vi "HighFrameRateRecording - DX cameras 2.vi"() -> ()   [LabVIEW 2010]
doc: "The LL Ring VI acquires images continuously and displays them in an image control using the low-level acquisition VIs. A ring initiates a continuous high-speed acquisition to multiple buffers and is appropriate for high-speed applications that perform processing on every image. Multiple buffers are useful when processing times vary depending on other applications and processing results .\n\nIMAQ Init initializes the device. IMAQ Configure List configures the buffer list with multiple buffers. IMAQ Create creates the image buffers. Call IMAQ Configure Buffer once for each buffer in the buffer list. IMAQ Start starts the acquisition, and IMAQ Extract Buffer ensures that the current image is not overwritten. An image control displays the image on the front panel. After exiting the loop, IMAQ Extract Buffer releases the last extracted buffer. IMAQ Close releases resources associated with the acquisition, and IMAQ Dispose frees the image buffer."
uses:
  <vilib>/vision/Avi.llb/IMAQ AVI2 Codec Path.ctl
  <vilib>/vision/driver/NI_Vision_Acquisition_Software.lvlib
  <vilib>/vision/driver/IMAQdx.llb/IMAQdx Acquisition Mode.ctl
  <vilib>/vision/driver/IMAQdx.llb/IMAQdx Buffer Number Mode.ctl
  <vilib>/vision/Avi.llb/IMAQ AVI2 Refnum.ctl
  <vilib>/userdefined/High Color/IMAQdx.ctl
panel:
  out "Frame Rate Graph":dbl(graph)=23.976023976023978
  out "FPS":dbl=24.7320692497939 format="%#.1f"
  in  "Camera Selection DX":T1="cam2"
  out "AVI Refnum":T2
  out "Video recording":bool
  in  "Record?":bool
  in  "codec index":i32=4
  out "codec":string="Motion JPEG (NI Vision)"
  in  "AVI File Path":path=path "E:/Video/24fps.avi"
  out "Processed Frames/s":dbl=23.976023976023978 format="%#.1g"
  in  "Stop":bool
  out "Saved Frames":i32
  out "Image":T3(plugin-control)
  # "ToDo:\n - add JSON output\n - andd indicator of _s# number"
  # "1.  Initialisation"
  # "Codec should be:\n\"Y800 Uncompressed Grey Scale\""
  # "Naming convention:\n - use the name above and add _s#.avi for videos\n - specs for saved videos is specified in name.json"
  # "2.  Recording"
  # "y"
  # "Record"
  # "x"
  # "Just Observe"
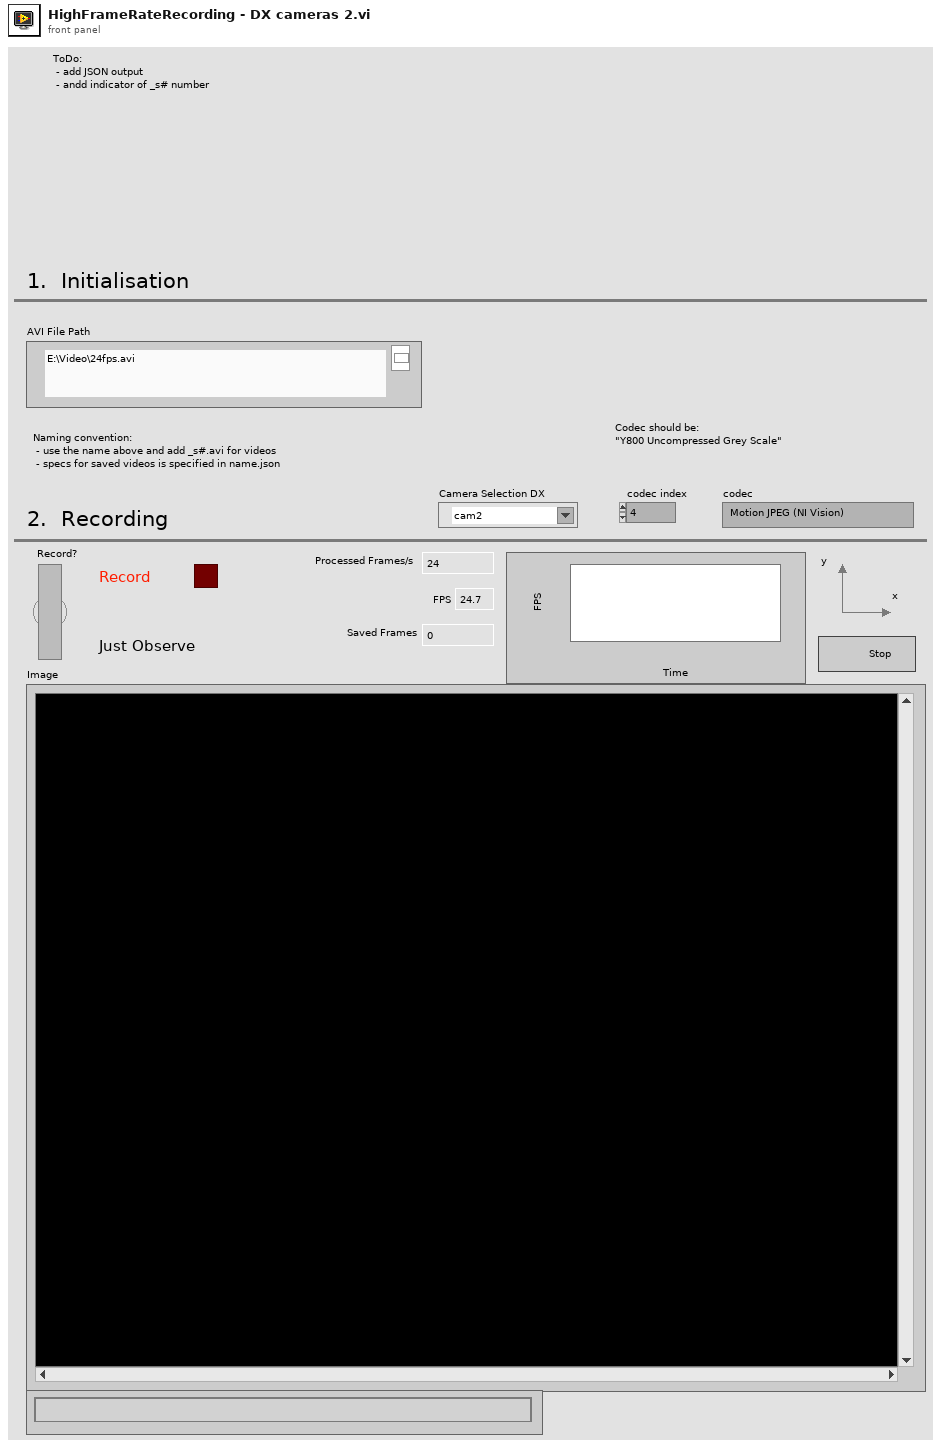
[diagram p1: front panel]
types:
  T1 = typedef "IMAQdx.ctl" = refnum<k21>
  T2 = typedef "IMAQ AVI2 Refnum.ctl" = refnum<k20>
  T3 = typedef "IMAQ Image.ctl" = refnum<image>
  T4 = typedef "NI_Vision_Acquisition_Software.lvlib/IMAQdx Acquisition Mode.ctl" = enum32{"One Shot", "Continuous"}
  T5 = typedef "IMAQ AVI2 Codec Path.ctl" = u32
  T6 = typedef "NI_Vision_Acquisition_Software.lvlib/IMAQdx Buffer Number Mode.ctl" = enum32{"Next", "Last", "Buffer Number", "Every", "Last New"}
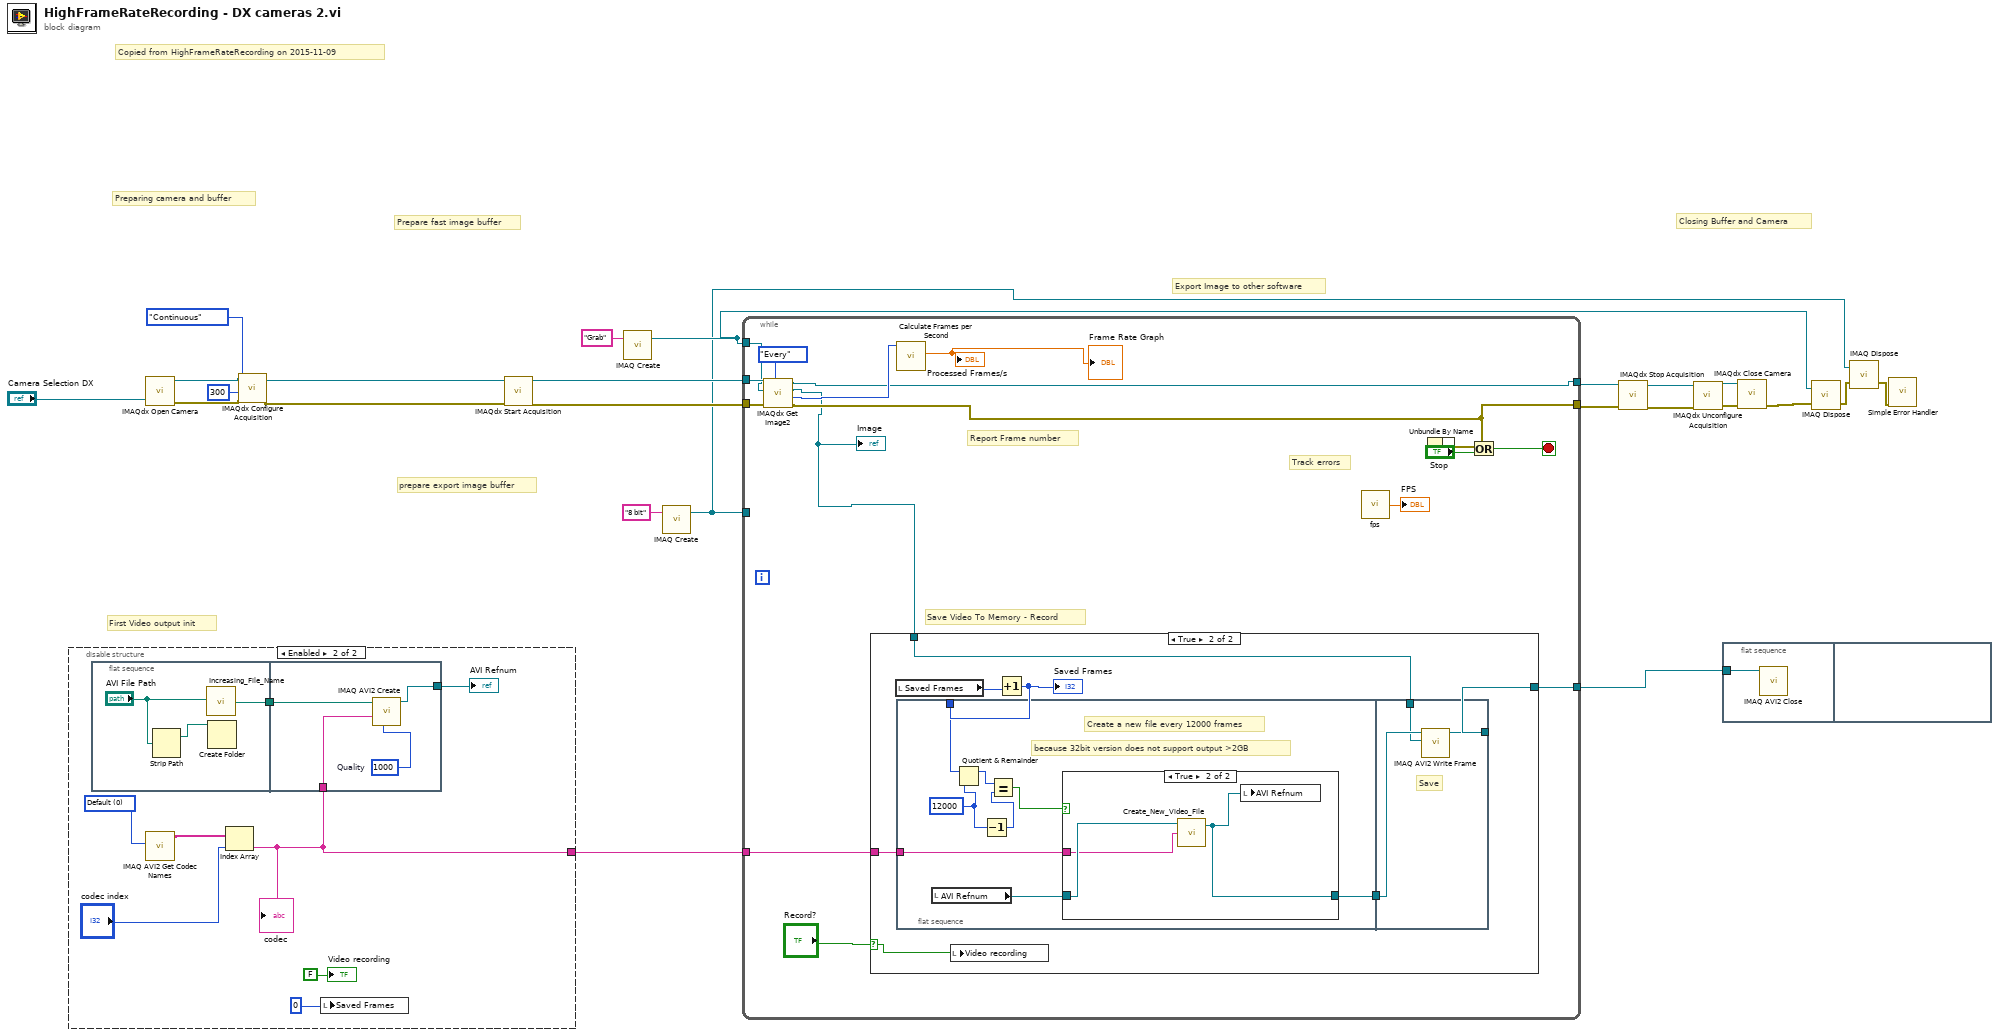
[diagram p0: block diagram]
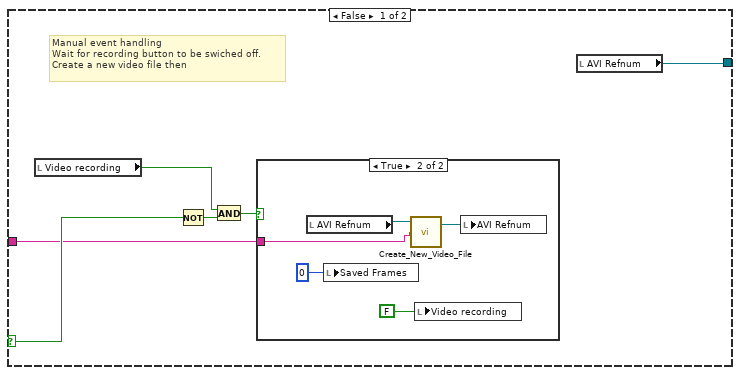
[diagram p3: hidden frame]
diagram:
  # "Copied from HighFrameRateRecording on 2015-11-09"
  # "Export Image to other software"
  # "prepare export image buffer"
  # "Prepare fast image buffer"
  # "First Video output init"
  # "Closing Buffer and Camera"
  # "Preparing camera and buffer"
  n1 = disable-structure shown="Enabled" {
    disable-tunnel: [_ w25] -> w23
    frame Disabled {
    }
    frame Enabled {
      w32 = T5 0 items=["Default", "System", "Built in Vision"] ("Codec Source")
      n2 = flat-sequence {
        tunnel: [w35] -> w27
        tunnel: w27 -> [w37]
        tunnel: [w38] -> w26
        tunnel: w25 -> [w36]
        frame #0 {
          n3 = Strip Path(path="AVI File Path") -> (stripped path=w34:path)  [unwired: 1 out]
          n4 = call "Increasing_File_Name.vi"("Base AVI  path"="AVI File Path") -> ("Final AVI path"=w35:path)
          n5 = Create Folder(path (use dialog)=w34) -> ()  [unwired: 2 in, 3 out]
        }
        frame #1 {
          w39 = 1000  # Quality
          n6 = call "IMAQ AVI2 Create"("Quality"=w39, "Codec"=w36, "AVI Path"=w37) -> ("AVI Refnum"=w38:T2)  [unwired: 7 in, 1 out]
        }
      }
      n7 = call "IMAQ AVI2 Get Codec Names"("Codec Source"=w32) -> ("Codec Names"=w31:string[])  [unwired: 9 in, 1 out]
      n8 = Index Array(array=w31, index="codec index") -> (element=w25:string)
      "codec" <- w25
      n9 = local write "Saved Frames"(0 ("Saved Frames")) -> ()
      "AVI Refnum" <- w26
      "Video recording" <- FALSE ("Video recording")
    }
  }
  n10 = call <vilib>:"IMAQdx Open Camera.vi"("Session In"="Camera Selection DX") -> ("error out"=w18:errorcluster, "Session Out"=w17:T1)  [unwired: 9 in]
  n11 = call <vilib>:"IMAQdx Configure Acquisition.vi"("error in"=w18, "Number of Buffers"=u32 300, "Continuous?"=IMAQdx_Acquisition_Mode."Continuous", "Session In"=w17) -> ("error out"=w11:errorcluster, "Session Out"=w12:T1)  [unwired: 6 in]
  n12 = call <vilib>:"IMAQdx Start Acquisition.vi"("error in"=w11, "Session In"=w12) -> ("error out"=w13:errorcluster, "Session Out"=w14:T1)  [unwired: 8 in]
  n13 = call "IMAQ Create"("Image Name"="Grab") -> ("New Image"=w19:T3)  [unwired: 3 in, 2 out]
  n14 = call "IMAQ Create"("Image Name"="8 bit") -> ("New Image"=w1:T3)  [unwired: 3 in, 2 out]
  n15 = while {
    tunnel: [w43] -> w6
    tunnel: [w45] -> w5
    tunnel: [w52] -> w24
    tunnel: w23 -> [w51]
    tunnel: w14 -> [w48]
    tunnel: w13 -> [w46]
    tunnel: w19 -> [w47]
    tunnel: w1 -> [_]
    stop <- w55 stop-if-true
    # "Track errors"
    # "Report Frame number"
    # "Save Video To Memory - Record"
    n16 = call <vilib>:"IMAQdx Get Image2.vi"("Buffer Number Mode (Next)"=IMAQdx_Buffer_Number_Mode."Every", "error in"=w46, "Image In"=w47, "Session In"=w48) -> ("error out"=w45:errorcluster, "Buffer Number Out"=w44:u32, "Image Out"=w41:T3, "Session Out"=w43:T1)  [unwired: 4 in]
    "Image" <- w41
    n17 = case shown="True" "Record?" {
      selector: "Record?" -> [w58 w68]
      tunnel: [w61 w71] -> w52
      tunnel: w41 -> [_ w69]
      tunnel: w51 -> [w56 w67]
      frame False {
        # "Manual event handling\nWait for recording button to be swiched off.\nCreate a new video file then"
        n18 = local read "Video recording"() -> (w57:bool)
        n19 = Not(x=w58) -> (.not. x?=w59:bool)
        n20 = And(x=w57, y=w59) -> (x .and. y?=w60:bool)
        n21 = case shown="True" w60 {
          tunnel: w56 -> [_ w62]
          frame False {
          }
          frame True {
            n22 = local read "AVI Refnum"() -> (w65:T2)
            n23 = local write "Saved Frames"(0 ("Saved Frames")) -> ()
            n24 = call "Create_New_Video_File.vi"("Codec"=w62, "AVI Refnum IN"=w65) -> ("AVI Refnum OUT"=w66:T2)  [unwired: 1 in, 1 out]
            n25 = local write "Video recording"(FALSE ("Video recording")) -> ()
            n26 = local write "AVI Refnum"(w66) -> ()
          }
        }
        n27 = local read "AVI Refnum"() -> (w61:T2)
      }
      frame True {
        n28 = local read "Saved Frames"() -> (w73:i32)
        n29 = flat-sequence {
          tunnel: w72 -> [w78]
          tunnel: [w75] -> w70
          tunnel: w67 -> [w74]
          tunnel: [w88] -> w71
          tunnel: w70 -> [w87]
          tunnel: w69 -> [w86]
          frame #0 {
            w80 = 12000 ("y")
            # "because 32bit version does not support output >2GB"
            # "Create a new file every 12000 frames"
            n30 = local read "AVI Refnum"() -> (w76:T2)
            n31 = Quotient & Remainder(x=w78, y=w80) -> (x-y*floor(x/y)=w81:i32)  [unwired: 1 out]
            n32 = Decrement(x=w80) -> (x-1=w79:i32)
            n33 = Equal?(x=w81, y=w79) -> (x = y?=w77:bool)
            n34 = case shown="True" w77 {
              tunnel: w76 -> [w82 w85]
              tunnel: [w82 w84] -> w75
              tunnel: w74 -> [_ w83]
              frame False {
              }
              frame True {
                n35 = call "Create_New_Video_File.vi"("Codec"=w83, "AVI Refnum IN"=w85) -> ("AVI Refnum OUT"=w84:T2)  [unwired: 1 in, 1 out]
                n36 = local write "AVI Refnum"(w84) -> ()
              }
            }
          }
          frame #1 {
            # "Save"
            n37 = call "IMAQ AVI2 Write Frame"("Image"=w86, "AVI Refnum"=w87) -> ("AVI Refnum (duplicate)"=w88:T2)  [unwired: 7 in, 2 out]
          }
        }
        n38 = local write "Video recording"(w68) -> ()
        n39 = Increment(x=w73) -> (x+1=w72:i32)
        "Saved Frames" <- w72
      }
    }
    n40 = call <vilib>:"Calculate Frames per Second.vi"("Buffer Number"=w44) -> ("Processed Frames/s"=→"Processed Frames/s" →"Frame Rate Graph":dbl)  [unwired: 8 in, 2 out]
    n41 = call "fps.vi"() -> ("FPS"=→"FPS":dbl)  [unwired: 1 in]
    n42 = Or(y="Stop") -> (x=w40:errorcluster, x .or. y?=w55:bool)
    n43 = Unbundle By Name(w45, w40) -> ()
  }
  n44 = call <vilib>:"IMAQdx Stop Acquisition.vi"("error in"=w5, "Session In"=w6) -> ("error out"=w7:errorcluster, "Session Out"=w8:T1)  [unwired: 8 in]
  n45 = call <vilib>:"IMAQdx Unconfigure Acquisition.vi"("error in"=w7, "Session In"=w8) -> ("error out"=w9:errorcluster, "Session Out"=w10:T1)  [unwired: 8 out]
  n46 = flat-sequence {
    tunnel: w24 -> [w89]
    frame #0 {
      n47 = call "IMAQ AVI2 Close"("AVI Refnum"=w89) -> ()  [unwired: 10 in, 1 out]
    }
    frame #1 {
    }
  }
  n48 = call <vilib>:"IMAQdx Close Camera.vi"("error in"=w9, "Session In"=w10) -> ("error out"=w21:errorcluster)  [unwired: 9 in]
  n49 = call "IMAQ Dispose"("Image"=w19, "error in (no error)"=w21) -> ("error out"=w3:errorcluster)  [unwired: 1 in, 3 out]
  n50 = call "IMAQ Dispose"("Image"=w1, "error in (no error)"=w3) -> ("error out"=w2:errorcluster)  [unwired: 1 in, 3 out]
  n51 = call <vilib>:"Simple Error Handler.vi"("error in (no error)"=w2) -> ()  [unwired: 1 in, 8 out]
